vi "TestAdd.vi"(11 "error in":errorcluster) -> (15 "error out":errorcluster)   [LabVIEW 2016, in "SimpleCalculatorTests.lvlib"]
doc: "The test script performs a series of addition operation and the output is asserted each time to the expected value"
uses:
  SimpleCalculatorTests.lvlib
  APIs/Stimulus/ControlValue/SetValueAuto.vi
  APIs/Assert/AssertControlValue/AlmostEqual.vi
  APIs/Stimulus/VI/CloseVI.vi
  Drona.lvlib
  <vilib>/addons/_JKI Toolkits/Caraya/classes/Test/Test.lvclass
  APIs/Stimulus/ControlValue/ControlValue.lvlib
  APIs/Stimulus/VI/VI.lvlib
  APIs/Assert/AssertControlValue/AssertControlValue.lvlib
panel:
  # "Drona Test Add"
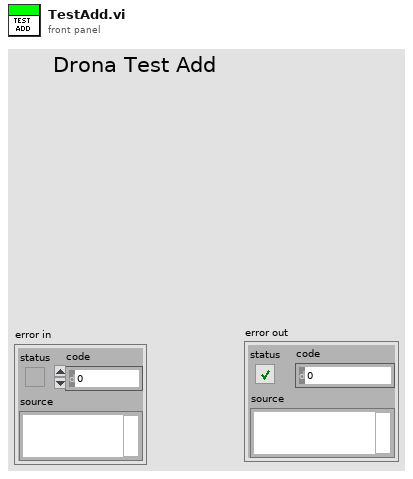
[diagram p1: front panel]
types:
  T1 = cluster{"Input 1":dbl, "Input 2":dbl, "Output":dbl}[]
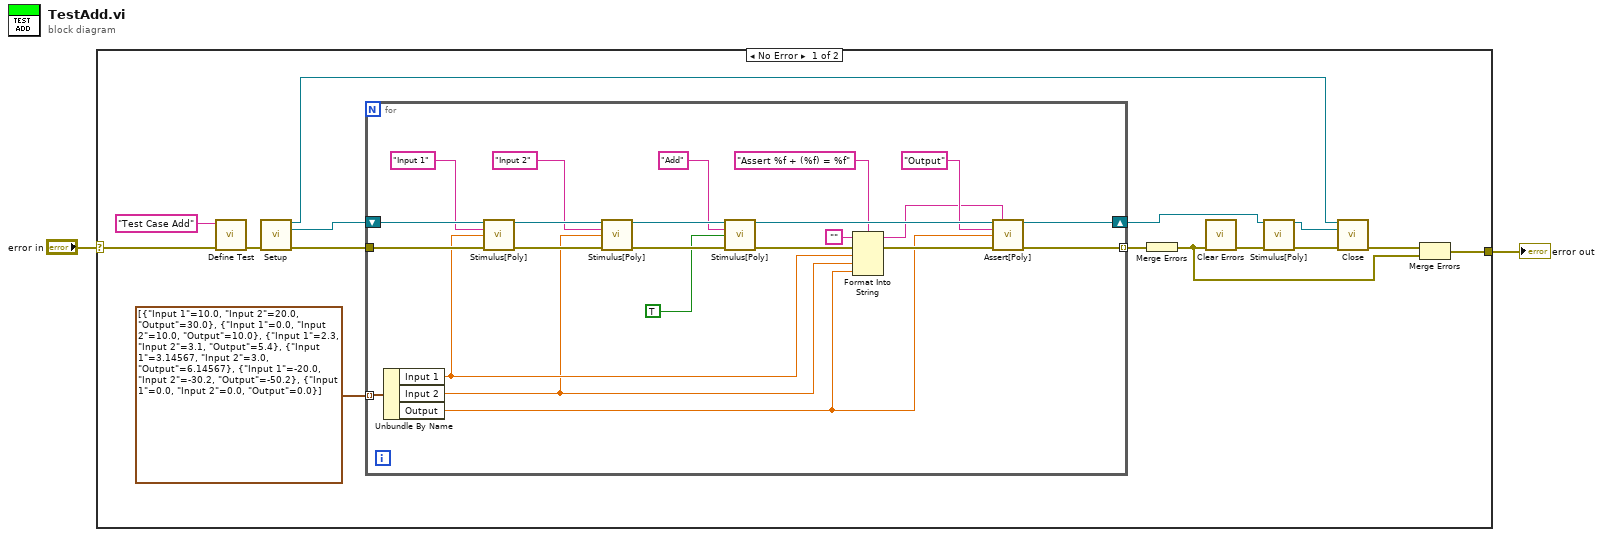
[diagram p0: block diagram]
diagram:
  n1 = case shown="No Error" "error in" {
    selector: "error in" -> [w3 w41]
    tunnel: [w5 w41] -> w2
    frame No Error {
      n2 = call <vilib>:"Define Test.vi"("error in (no error)"=w3, "Label (VI Title)"="Test Case Add") -> ("error out"=w13:errorcluster)  [unwired: 8 in, 1 out]
      n3 = call "Setup.vi"("error in"=w13) -> ("Application Ref"=w15:refnum<vi>, "VI Reference Out"=w17:refnum<vi>, "error out"=w16:errorcluster)  [unwired: 12 in]
      n4 = for {
        shift-right: [w28] -> w9
        shift-left: w17 -> [w40]
        tunnel: T1 [{"Input 1"=10.0, "Input 2"=20.0, "Output"=30.0}, {"Input 1"=0.0, "Input 2"=10.0, "Output"=10.0}, {"Input 1"=2.3, "Input 2"=3.1, "Output"=5.4}, {"Input 1"=3.14567, "Input 2"=3.0, "Output"=6.14567}, {"Input 1"=-20.0, "Input 2"=-30.2, "Output"=-50.2}, {"Input 1"=0.0, "Input 2"=0.0, "Output"=0.0}] -> [w26] mode=indexing
        tunnel: w16 -> [w39]
        tunnel: [w30] -> w14 mode=indexing
        n5 = Unbundle By Name(w26) -> ("Input 1"=w23:dbl, "Input 2"=w22:dbl, "Output"=w21:dbl)
        n6 = call-poly "Stimulus[Poly].vi"("VI Reference In"=w40, "Control Path"="Input 1", "Value (Signaling)"=w23, "error in"=w39) -> ("VI Reference Out"=w36:refnum<vi>, "error out"=w37:errorcluster)  [unwired: 10 in]
        n7 = call-poly "Stimulus[Poly].vi"("VI Reference In"=w36, "Control Path"="Input 2", "Value (Signaling)"=w22, "error in"=w37) -> ("VI Reference Out"=w34:refnum<vi>, "error out"=w33:errorcluster)  [unwired: 10 in]
        n8 = call-poly "Stimulus[Poly].vi"("VI Reference In"=w34, "Control Path"="Add", "Value (Signaling)"=TRUE, "error in"=w33) -> ("VI Reference Out"=w29:refnum<vi>, "error out"=w31:errorcluster)  [unwired: 10 in]
        n9 = Format Into String(format string="Assert %f + (%f) = %f", initial string="", error in=w31, w23, w22, w21) -> (resulting string=w20:string, error out=w25:errorcluster)
        n10 = call-poly "Assert[Poly].vi"("VI Reference In"=w29, "Test Label"=w20, "Control Path"="Output", "Control Value"=w21, "Error In"=w25) -> ("VI Reference Out"=w28:refnum<vi>, "Error Out"=w30:errorcluster)  [unwired: 8 in, 1 out]
      }
      n11 = Merge Errors(w14) -> (w4:errorcluster)
      n12 = call <vilib>:"Clear Errors.vi"("error in (no error)"=w4) -> ("error out"=w10:errorcluster)  [unwired: 5 in, 1 out]
      n13 = call-poly "Stimulus[Poly].vi"("VI Reference In"=w9, "error in"=w10) -> ("VI Reference Out"=w8:refnum<vi>, "error out"=w7:errorcluster)  [unwired: 12 in]
      n14 = call "Close.vi"("Application Ref"=w15, "VI Reference"=w8, "error in"=w7) -> ("error out"=w6:errorcluster)  [unwired: 12 in]
      n15 = Merge Errors(w6, w4) -> (w5:errorcluster)
    }
    frame Error {
    }
  }
  "error out" <- w2
